vi "connectUDP.vi"(0 "port or service name NOT USED":u16) -> (1 "fast ID (h)":refnum<k16>, 2 "slow ID (h)":refnum<k16>, 3 "connections (hidden)":variant[](array[variant])=[variant(refnum<k16> refnum), variant(refnum<k16> refnum)], 4 "local Port":u16=65401)   [LabVIEW 2018]
panel:
  out "error out":errorcluster
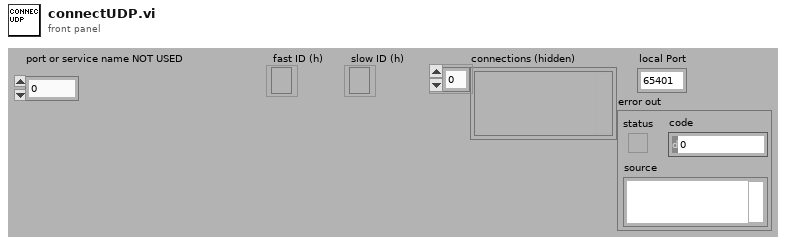
[diagram p1: front panel]
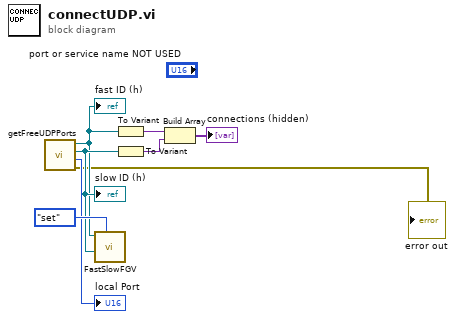
[diagram p0: block diagram]
diagram:
  n1 = call "getFreeUDPPorts.vi"() -> ("error out"=→"error out":errorcluster, "local Port"=→"local Port":u16, "slow"=w4:refnum<k16>, "fast"=w3:refnum<k16>)  [unwired: 8 in]
  "fast ID (h)" <- w3
  "slow ID (h)" <- w4
  n2 = call "FastSlowFGV.vi"("Command"=enum16{"get", "set", "init"}."set", "slow ID"=w4, "fast ID"=w3) -> ()  [unwired: 7 in, 2 out]
  n3 = To Variant(anything=w3) -> (Variant=w6:variant)
  n4 = To Variant(anything=w4) -> (Variant=w5:variant)
  n5 = Build Array(w6, w5) -> (→"connections (hidden)":variant[])
